vi "1_StartStopServer.vi"(6 "T:start":bool, 8 "error in (no error)":errorcluster caption="错误输入（无错误）", 9 "remote port (80)":u16=1883, 10 "address (localhost)":string="localhost", 11 "MQTT_Server_Actor 输入":refnum<class "MQTT_Server_Actor.lvclass">) -> (0 "error out":errorcluster caption="错误输出", 3 "MQTT_Server_Actor 输出":refnum<class "MQTT_Server_Actor.lvclass">)   [LabVIEW 2018, in "MQTT_Server_Actor.lvlib" / "MQTT_Server_Actor.lvclass"]
uses:
  MQTT_Server_Actor.lvclass
  StartServer.ctl
  MQTT_Server_Actor.lvclass/MQTT_Server_Actor.ctl
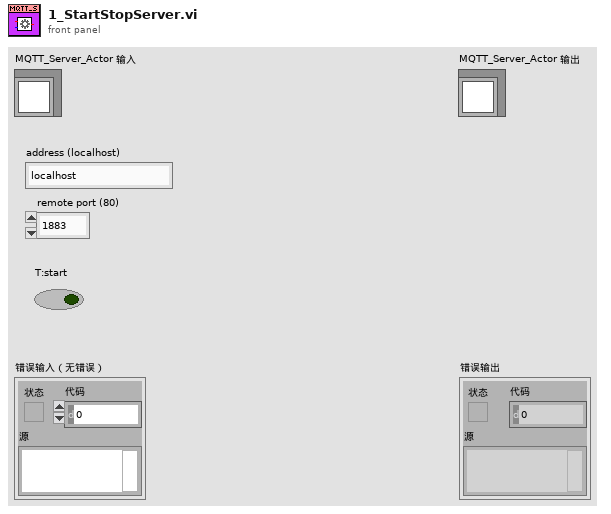
[diagram p1: front panel]
types:
  T1 = typedef "MQTT_Server_Actor.lvlib/MQTT_Server_Actor.lvclass/StartServer.ctl" = cluster{"address (localhost)":string, "remote port (80)":u16, "StartServer":bool}
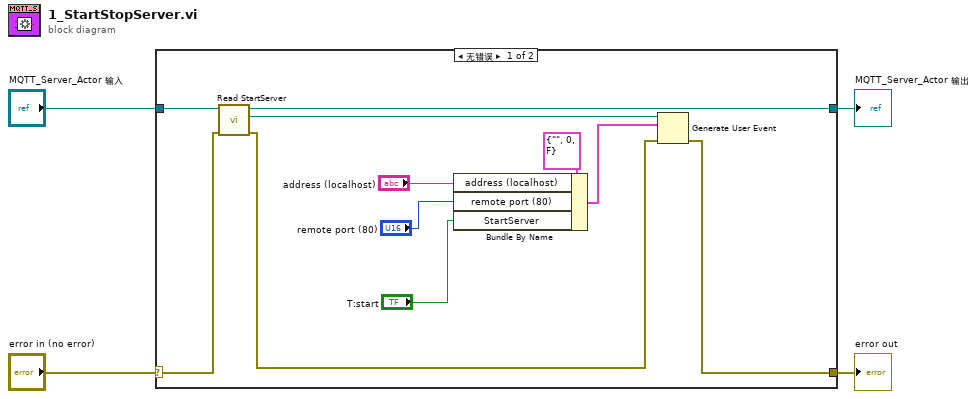
[diagram p0: block diagram]
diagram:
  n1 = case shown="无错误" "error in (no error)" {
    selector: "error in (no error)" -> [w13 w17]
    tunnel: [w10 w17] -> w3
    tunnel: [w14 w16] -> w1
    tunnel: "MQTT_Server_Actor 输入" -> [w15 w16]
    frame No Error {
      n2 = call "Read StartServer.vi"("error in (no error)"=w13, "MQTT_Server_Actor输入"=w15) -> ("error out"=w11:errorcluster, "StartServer"=w12:refnum<user-event>, "MQTT_Server_Actor输出"=w14:refnum<class "MQTT_Server_Actor.lvclass">)  [unwired: 7 in]
      n3 = Bundle By Name(cluster=T1 {"address (localhost)"="", "remote port (80)"=0, "StartServer"=FALSE} ("事件数据"), "address (localhost)"="address (localhost)", "remote port (80)"="remote port (80)", "StartServer"="T:start") -> (w8:T1)
      n4 = Generate User Event(user event=w12, event data cluster=w8, error in=w11) -> (error out=w10:errorcluster)  [unwired: 1 in, 1 out]
    }
    frame Error {
    }
  }
  "error out" <- w3
  "MQTT_Server_Actor 输出" <- w1
